vi "Image Averaging.vi"() -> ()   [LabVIEW 2014]
doc: "This example shows how to use image averaging to improve the signal/noise ratio of noisy images."
uses:
  <vilib>/vision/NI_Vision_Development_Module.lvlib
panel:
  out "Images Accumulated":i32
  out "Image Source":T1(plugin-control)
  out "Averaged Image":T1(plugin-control)
  # "Overview: Demonstrates how to use arithmetic operators to average images and reduce the image noise level.\nRequirements: NI Vision Development Module\nInstructions: Run the VI."
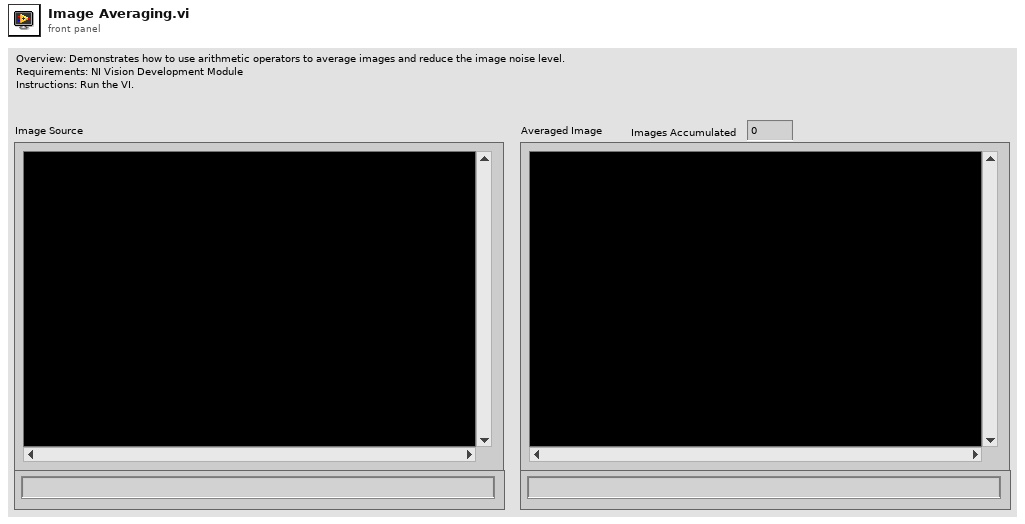
[diagram p1: front panel]
types:
  T1 = typedef "IMAQ Image.ctl" = refnum<image>
  T2 = typedef "Image Type" = u32
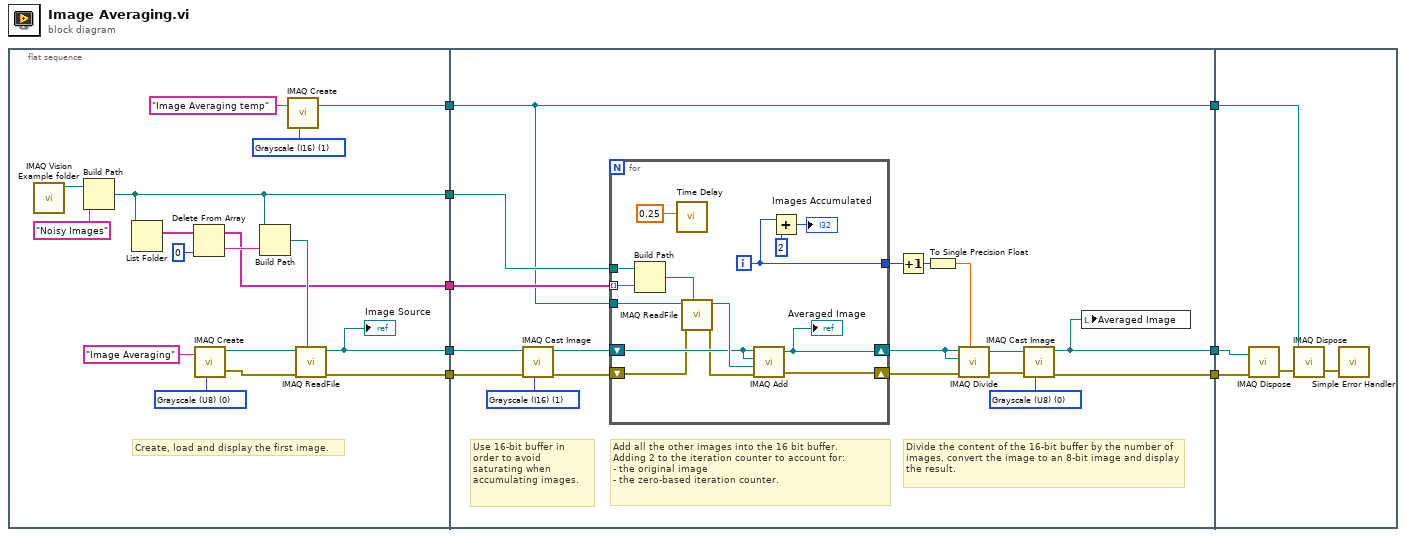
[diagram p0: block diagram]
diagram:
  n1 = flat-sequence {
    tunnel: [w10] -> w8
    tunnel: [w19] -> w7
    tunnel: [w18] -> w6
    tunnel: [w15] -> w5
    tunnel: [w13] -> w2
    tunnel: w8 -> [w43]
    tunnel: w7 -> [w36]
    tunnel: w6 -> [w34]
    tunnel: w5 -> [w33]
    tunnel: [w33] -> w4
    tunnel: [w32] -> w3
    tunnel: w2 -> [w31]
    tunnel: [w26] -> w1
    tunnel: w4 -> [w62]
    tunnel: w3 -> [w61]
    tunnel: w1 -> [w60]
    frame #0 {
      w17 = T2 1 items=["Grayscale (U8)", "Grayscale (I16)", "Grayscale (SGL)", "Complex (CSG)", "RGB (U32)", "HSL (U32)", "RGB (U64)", "Grayscale (U16)"] ("Image Type")
      w23 = T2 0 items=["Grayscale (U8)", "Grayscale (I16)", "Grayscale (SGL)", "Complex (CSG)", "RGB (U32)", "HSL (U32)", "RGB (U64)", "Grayscale (U16)"] ("Image Type")
      # "Create, load and display the first image."
      n2 = call "IMAQ Vision Example folder.vi"() -> ("Example Image Path"=w22:path)  [unwired: 11 in]
      n3 = Build Path(base path=w22, name or relative path="Noisy Images") -> (appended path=w18:path)
      n4 = List Folder(path=w18) -> (filenames=w9:string[])  [unwired: 3 in, 3 out]
      n5 = Delete From Array(array=w9, index=0) -> (deleted portion=w11:string, array with subset deleted=w10:string[])  [unwired: 1 in]
      n6 = call "IMAQ Create"("Image Name"="Image Averaging", "Image Type"=w23) -> ("New Image"=w25:T1, "error out"=w14:errorcluster)  [unwired: 3 in]
      n7 = Build Path(base path=w18, name or relative path=w11) -> (appended path=w24:path)
      n8 = call "IMAQ Create"("Image Name"="Image Averaging temp", "Image Type"=w17) -> ("New Image"=w15:T1)  [unwired: 3 in, 1 out]
      n9 = call "IMAQ ReadFile"("File Path"=w24, "error in (no error)"=w14, "Image"=w25) -> ("error out"=w13:errorcluster, "Image Out"=w19:T1)  [unwired: 4 in, 3 out]
      "Image Source" <- w19
    }
    frame #1 {
      w37 = T2 1 items=["Grayscale (U8)", "Grayscale (I16)", "Grayscale (SGL)", "Complex (CSG)", "RGB (U32)", "HSL (U32)", "RGB (U64)", "Grayscale (U16)"] ("Image Type")
      w38 = T2 0 items=["Grayscale (U8)", "Grayscale (I16)", "Grayscale (SGL)", "Complex (CSG)", "RGB (U32)", "HSL (U32)", "RGB (U64)", "Grayscale (U16)"] ("Image Type")
      # "Add all the other images into the 16 bit buffer.\nAdding 2 to the iteration counter to account for: \n- the original image\n- the zero-based iteration counter."
      # "Use 16-bit buffer in order to avoid saturating when accumulating images."
      # "Divide the content of the 16-bit buffer by the number of images, convert the image to an 8-bit image and display the result."
      n10 = call "IMAQ Cast Image"("Image Type"=w37, "error in (no error)"=w31, "Image Src"=w36) -> ("error out"=w29:errorcluster, "Image Dst Out"=w35:T1)  [unwired: 7 in]
      n11 = for {
        tunnel: w34 -> [w57]
        tunnel: w43 -> [w56] mode=indexing
        tunnel: w33 -> [w54]
        shift-right: [w51] -> w41
        shift-left: w35 -> [w52]
        tunnel: [w46] -> w40
        shift-right: [w50] -> w28
        shift-left: w29 -> [w49]
        i -> [w46]
        n12 = Build Path(base path=w57, name or relative path=w56) -> (appended path=w55:path)
        n13 = call "Time Delay"("Delay Time (s)"=0.25) -> ()  [unwired: 10 in, 1 out]
        n14 = call "IMAQ ReadFile"("File Path"=w55, "error in (no error)"=w49, "Image"=w54) -> ("error out"=w48:errorcluster, "Image Out"=w53:T1)  [unwired: 4 in, 3 out]
        n15 = call "IMAQ Add"("Image Src A"=w52, "Image Dst"=w52, "Image Src B"=w53, "error in (no error)"=w48) -> ("Image Dst Out"=w51:T1, "error out"=w50:errorcluster)  [unwired: 3 in]
        "Averaged Image" <- w51
        n16 = Add(x=w46, y=2) -> (x+y=→"Images Accumulated":i32)
      }
      n17 = Increment(x=w40) -> (x+1=w39:i32)
      n18 = To Single Precision Float(number=w39) -> (single precision float=w30:sgl)
      n19 = call "IMAQ Divide"("Image Src A"=w41, "Constant"=w30, "Image Dst"=w41, "error in (no error)"=w28) -> ("Image Dst Out"=w42:T1, "error out"=w27:errorcluster)  [unwired: 3 in]
      n20 = call "IMAQ Cast Image"("Image Type"=w38, "error in (no error)"=w27, "Image Src"=w42) -> ("error out"=w26:errorcluster, "Image Dst Out"=w32:T1)  [unwired: 7 in]
      n21 = local write "Averaged Image"(w32) -> ()
    }
    frame #2 {
      n22 = call "IMAQ Dispose"("Image"=w61, "error in (no error)"=w60) -> ("error out"=w59:errorcluster)  [unwired: 4 in]
      n23 = call "IMAQ Dispose"("Image"=w62, "error in (no error)"=w59) -> ("error out"=w58:errorcluster)  [unwired: 4 in]
      n24 = call <vilib>:"Simple Error Handler.vi"("error in (no error)"=w58) -> ()  [unwired: 4 in, 5 out]
    }
  }
